vi "Weather Parse Test.vi"() -> ()   [LabVIEW 2020, in "CDM-Config.lvlib"] (continued)
eferences\": [\n                    {\n                        \"@id\": \"https://api.weather.gov/alerts/urn:oid:2.49.0.1.840.0.e016f252f56054b547b3ac73b3419f6e51da412e.001.4\",\n                        \"identifier\": \"urn:oid:2.49.0.1.840.0.e016f252f56054b547b3ac73b3419f6e51da412e.001.4\",\n                        \"sender\": \"w-nws.webmaster@noaa.gov\",\n                        \"sent\": \"2025-12-03T03:23:00-05:00\"\n                    },\n                    {\n                        \"@id\": \"https://api.weather.gov/alerts/urn:oid:2.49.0.1.840.0.e016f252f56054b547b3ac73b3419f6e51da412e.003.3\",\n                        \"identifier\": \"urn:oid:2.49.0.1.840.0.e016f252f56054b547b3ac73b3419f6e51da412e.003.3\",\n                        \"sender\": \"w-nws.webmaster@noaa.gov\",\n                        \"sent\": \"2025-12-03T03:23:00-05:00\"\n                    }\n                ],\n                \"sent\": \"2025-12-03T10:58:00-05:00\",\n                \"effective\": \"2025-12-03T10:58:00-05:00\",\n                \"onset\": \"2025-12-03T19:00:00-05:00\",\n                \"expires\": \"2025-12-03T23:00:00-05:00\",\n                \"ends\": \"2025-12-04T07:00:00-05:00\",\n                \"status\": \"Actual\",\n                \"messageType\": \"Update\",\n                \"category\": \"Met\",\n                \"severity\": \"Severe\",\n                \"certainty\": \"Likely\",\n                \"urgency\": \"Expected\",\n                \"event\": \"Heavy Freezing Spray Warning\",\n                \"sender\": \"w-nws.webmaster@noaa.gov\",\n                \"senderName\": \"NWS Marquette MI\",\n                \"headline\": \"Heavy Freezing Spray Warning issued December 3 at 10:58AM EST until December 4 at 7:00AM EST by NWS Marquette MI\",\n                \"description\": \"* WHAT...For the Gale Warning, northwest winds 25 to 30 kt with\\ngusts up to 40 kt and waves 8 to 13 ft occurring. For the\\nHeavy Freezing Spray Warning, heavy freezing spray at a rate\\nof 2 cm per hour or greater expected, and may rapidly\\naccumulate on vessels.\\n\\n* WHERE...Eagle River to Manitou Island MI, Lake Superior from\\nUpper Entrance to Portage Canal to Manitou Island MI 5NM off\\nshore to the US/Canadian Border and Lake Superior East of a\\nline from Manitou Island to Marquette MI and West of a line\\nfrom Grand Marais MI to the US/Canadian Border Beyond 5NM from\\nshore.\\n\\n* WHEN...For the Gale Warning, until 7 AM EST Thursday. For the\\nHeavy Freezing Spray Warning, from 7 PM this evening to 7 AM\\nEST Thursday.\\n\\n* IMPACTS...Operating a vessel in heavy freezing spray is\\nhazardous. Freezing spray may render mechanical and electronic\\ncomponents inoperative. Rapid ice accretion on decks and\\nsuperstructures may result in a catastrophic loss of\\nstability. Strong winds will cause hazardous waves which could\\ncapsize or damage vessels and reduce visibility.\",\n                \"instruction\": \"Mariners should prepare for dangerous accumulation of ice on\\ntheir vessel. If possible, remain in port, avoid the warning area\\nor conduct mitigation.\\n\\nMariners should alter plans to avoid these hazardous conditions.\\nRemain in port, seek safe harbor, alter course, and/or secure the\\nvessel for hazardous conditions.\",\n                \"response\": \"Avoid\",\n                \"parameters\": {\n                    \"AWIPSidentifier\": [\n                        \"MWWMQT\"\n                    ],\n                    \"WMOidentifier\": [\n                        \"WHUS73 KMQT 031558\"\n                    ],\n                    \"NWSheadline\": [\n                        \"GALE WARNING REMAINS IN EFFECT UNTIL 7 AM EST THURSDAY... ...HEAVY FREEZING SPRAY WARNING REMAINS IN EFFECT FROM 7 PM THIS EVENING TO 7 AM EST THURSDAY\"\n                    ],\n                    \"BLOCKCHANNEL\": [\n                        \"EAS\",\n                        \"NWEM\",\n                        \"CMAS\"\n                    ],\n                    \"VTEC\": [\n                        \"/O.CON.KMQT.UP.W.0017.251204T0000Z-251204T1200Z/\"\n                    ],\n                    \"eventEndingTime\": [\n                        \"2025-12-04T07:00:00-05:00\"\n                    ]\n                },\n                \"scope\": \"Public\",\n                \"code\": \"IPAWSv1.0\",\n                \"language\": \"en-US\",\n                \"web\": \"http://www.weather.gov\",\n                \"eventCode\": {\n                    \"SAME\": [\n                        \"NWS\"\n                    ],\n                    \"NationalWeatherService\": [\n                        \"UPW\"\n                    ]\n                }\n            }\n        },\n        {\n            \"id\": \"https://api.weather.gov/alerts/urn:oid:2.49.0.1.840.0.cfec64fd36b2ac790d0ebe73b8c20f8dfc3ec5cb.003.1\",\n            \"type\": \"Feature\",\n            \"geometry\": null,\n            \"properties\": {\n                \"@id\": \"https://api.weather.gov/alerts/urn:oid:2.49.0.1.840.0.cfec64fd36b2ac790d0ebe73b8c20f8dfc3ec5cb.003.1\",\n                \"@type\": \"wx:Alert\",\n                \"id\": \"urn:oid:2.49.0.1.840.0.cfec64fd36b2ac790d0ebe73b8c20f8dfc3ec5cb.003.1\",\n                \"areaDesc\": \"Black River To Ontonagon MI\",\n                \"geocode\": {\n                    \"SAME\": [\n                        \"091241\"\n                    ],\n                    \"UGC\": [\n                        \"LSZ241\"\n                    ]\n                },\n                \"affectedZones\": [\n                    \"https://api.weather.gov/zones/forecast/LSZ241\"\n                ],\n                \"references\": [\n                    {\n                        \"@id\": \"https://api.weather.gov/alerts/urn:oid:2.49.0.1.840.0.e016f252f56054b547b3ac73b3419f6e51da412e.004.1\",\n                        \"identifier\": \"urn:oid:2.49.0.1.840.0.e016f252f56054b547b3ac73b3419f6e51da412e.004.1\",\n                        \"sender\": \"w-nws.webmaster@noaa.gov\",\n                        \"sent\": \"2025-12-03T03:23:00-05:00\"\n                    }\n                ],\n                \"sent\": \"2025-12-03T10:58:00-05:00\",\n                \"effective\": \"2025-12-03T10:58:00-05:00\",\n                \"onset\": \"2025-12-03T10:58:00-05:00\",\n                \"expires\": \"2025-12-03T23:00:00-05:00\",\n                \"ends\": \"2025-12-03T16:00:00-05:00\",\n                \"status\": \"Actual\",\n                \"messageType\": \"Update\",\n                \"category\": \"Met\",\n                \"severity\": \"Minor\",\n                \"certainty\": \"Likely\",\n                \"urgency\": \"Expected\",\n                \"event\": \"Small Craft Advisory\",\n                \"sender\": \"w-nws.webmaster@noaa.gov\",\n                \"senderName\": \"NWS Marquette MI\",\n                \"headline\": \"Small Craft Advisory issued December 3 at 10:58AM EST until December 3 at 4:00PM EST by NWS Marquette MI\",\n                \"description\": \"* WHAT...For the Small Craft Advisory, northwest winds 20 to 25\\nkt with gusts up to 30 kt and waves around 7 ft occurring. For\\nthe Gale Warning, northwest winds around 25 kt with gusts up\\nto 35 kt and waves 7 to 9 ft expected.\\n\\n* WHERE...Black River to Ontonagon MI.\\n\\n* WHEN...For the Small Craft Advisory, until 4 PM EST /3 PM CST/\\nthis afternoon. For the Gale Warning, from 4 PM EST /3 PM CST/\\nthis afternoon to 1 AM EST /midnight CST/ Thursday.\\n\\n* IMPACTS...Strong winds will cause hazardous waves which could\\ncapsize or damage vessels and reduce visibility.\",\n                \"instruction\": \"Mariners should alter plans to avoid these hazardous conditions.\\nRemain in port, seek safe harbor, alter course, and/or secure the\\nvessel for hazardous conditions.\",\n                \"response\": \"Avoid\",\n                \"parameters\": {\n                    \"AWIPSidentifier\": [\n                        \"MWWMQT\"\n                    ],\n                    \"WMOidentifier\": [\n                        \"WHUS73 KMQT 031558\"\n                    ],\n                    \"NWSheadline\": [\n                        \"SMALL CRAFT ADVISORY REMAINS IN EFFECT UNTIL 4 PM EST /3 PM CST/ THIS AFTERNOON... ...GALE WARNING REMAINS IN EFFECT FROM 4 PM EST /3 PM CST/ THIS AFTERNOON TO 1 AM EST /MIDNIGHT CST/ THURSDAY\"\n                    ],\n                    \"BLOCKCHANNEL\": [\n                        \"EAS\",\n                        \"NWEM\",\n                        \"CMAS\"\n                    ],\n                    \"VTEC\": [\n                        \"/O.CON.KMQT.SC.Y.0191.000000T0000Z-251203T2100Z/\"\n                    ],\n                    \"eventEndingTime\": [\n                        \"2025-12-03T16:00:00-05:00\"\n                    ],\n                    \"expiredReferences\": [\n                        \"w-nws.webmaster@noaa.gov,urn:oid:2.49.0.1.840.0.012a713e44cf33f321dde7a7dd606454111e7dbb.001.1,2025-12-02T22:29:00-05:00 w-nws.webmaster@noaa.gov,urn:oid:2.49.0.1.840.0.74d44099106d0ecd40f7d2a62c56231069593ff3.001.1,2025-12-02T14:53:00-05:00 w-nws.webmaster@noaa.gov,urn:oid:2.49.0.1.840.0.747dd730e6a8b18ac9024c3c055a74162144c3ca.001.1,2025-12-02T10:16:00-05:00 w-nws.webmaster@noaa.gov,urn:oid:2.49.0.1.840.0.9d4c1194cc60ce916e8ebdf8581f4113872ed30b.001.1,2025-12-02T03:21:00-05:00\"\n                    ]\n                },\n                \"scope\": \"Public\",\n                \"code\": \"IPAWSv1.0\",\n                \"language\": \"en-US\",\n                \"web\": \"http://www.weather.gov\",\n                \"eventCode\": {\n                    \"SAME\": [\n                        \"NWS\"\n                    ],\n                    \"NationalWeatherService\": [\n                        \"SCY\"\n                    ]\n                }\n            }\n        },\n        {\n            \"id\": \"https://api.weather.gov/alerts/urn:oid:2.49.0.1.840.0.cfec64fd36b2ac790d0ebe73b8c20f8dfc3ec5cb.003.2\",\n            \"type\": \"Feature\",\n            \"geometry\": null,\n            \"properties\": {\n                \"@id\": \"https://api.weather.gov/alerts/urn:oid:2.49.0.1.840.0.cfec64fd36b2ac790d0ebe73b8c20f8dfc3ec5cb.003.2\",\n                \"@type\": \"wx:Alert\",\n                \"id\": \"urn:oid:2.49.0.1.840.0.cfec64fd36b2ac790d0ebe73b8c20f8dfc3ec5cb.003.2\",\n                \"areaDesc\": \"Black River To Ontonagon MI\",\n                \"geocode\": {\n                    \"SAME\": [\n                        \"091241\"\n                    ],\n                    \"UGC\": [\n                        \"LSZ241\"\n                    ]\n                },\n                \"affectedZones\": [\n                    \"https://api.weather.gov/zones/forecast/LSZ241\"\n                ],\n                \"references\": [\n                    {\n                        \"@id\": \"https://api.weather.gov/alerts/urn:oid:2.49.0.1.840.0.e016f252f56054b547b3ac73b3419f6e51da412e.004.3\",\n                        \"identifier\": \"urn:oid:2.49.0.1.840.0.e016f252f56054b547b3ac73b3419f6e51da412e.004.3\",\n                        \"sender\": \"w-nws.webmaster@noaa.gov\",\n                        \"sent\": \"2025-12-03T03:23:00-05:00\"\n                    }\n                ],\n                \"sent\": \"2025-12-03T10:58:00-05:00\",\n                \"effective\": \"2025-12-03T10:58:00-05:00\",\n                \"onset\": \"2025-12-03T16:00:00-05:00\",\n                \"expires\": \"2025-12-03T23:00:00-05:00\",\n                \"ends\": \"2025-12-04T01:00:00-05:00\",\n                \"status\": \"Actual\",\n                \"messageType\": \"Update\",\n                \"category\": \"Met\",\n                \"severity\": \"Moderate\",\n                \"certainty\": \"Likely\",\n                \"urgency\": \"Expected\",\n                \"event\": \"Gale Warning\",\n                \"sender\": \"w-nws.webmaster@noaa.gov\",\n                \"senderName\": \"NWS Marquette MI\",\n                \"headline\": \"Gale Warning issued December 3 at 10:58AM EST until December 4 at 1:00AM EST by NWS Marquette MI\",\n                \"description\": \"* WHAT...For the Small Craft Advisory, northwest winds 20 to 25\\nkt with gusts up to 30 kt and waves around 7 ft occurring. For\\nthe Gale Warning, northwest winds around 25 kt with gusts up\\nto 35 kt and waves 7 to 9 ft expected.\\n\\n* WHERE...Black River to Ontonagon MI.\\n\\n* WHEN...For the Small Craft Advisory, until 4 PM EST /3 PM CST/\\nthis afternoon. For the Gale Warning, from 4 PM EST /3 PM CST/\\nthis afternoon to 1 AM EST /midnight CST/ Thursday.\\n\\n* IMPACTS...Strong winds will cause hazardous waves which could\\ncapsize or damage vessels and reduce visibility.\",\n                \"instruction\": \"Mariners should alter plans to avoid these hazardous conditions.\\nRemain in port, seek safe harbor, alter course, and/or secure the\\nvessel for hazardous conditions.\",\n                \"response\": \"Avoid\",\n                \"parameters\": {\n                    \"AWIPSidentifier\": [\n                        \"MWWMQT\"\n                    ],\n                    \"WMOidentifier\": [\n                        \"WHUS73 KMQT 031558\"\n                    ],\n                    \"NWSheadline\": [\n                        \"SMALL CRAFT ADVISORY REMAINS IN EFFECT UNTIL 4 PM EST /3 PM CST/ THIS AFTERNOON... ...GALE WARNING REMAINS IN EFFECT FROM 4 PM EST /3 PM CST/ THIS AFTERNOON TO 1 AM EST /MIDNIGHT CST/ THURSDAY\"\n                    ],\n                    \"BLOCKCHANNEL\": [\n                        \"EAS\",\n                        \"NWEM\",\n                        \"CMAS\"\n                    ],\n                    \"VTEC\": [\n                        \"/O.CON.KMQT.GL.W.0057.251203T2100Z-251204T0600Z/\"\n                    ],\n                    \"eventEndingTime\": [\n                        \"2025-12-04T01:00:00-05:00\"\n                    ]\n                },\n                \"scope\": \"Public\",\n                \"code\": \"IPAWSv1.0\",\n                \"language\": \"en-US\",\n                \"web\": \"http://www.weather.gov\",\n                \"eventCode\": {\n                    \"SAME\": [\n                        \"NWS\"\n                    ],\n                    \"NationalWeatherService\": [\n                        \"GLW\"\n                    ]\n                }\n            }\n        },\n        {\n            \"id\": \"https://api.weather.gov/alerts/urn:oid:2.49.0.1.840.0.cfec64fd36b2ac790d0ebe73b8c20f8dfc3ec5cb.006.1\",\n            \"type\": \"Feature\",\n            \"geometry\": null,\n            \"properties\": {\n                \"@id\": \"https://api.weather.gov/alerts/urn:oid:2.49.0.1.840.0.cfec64fd36b2ac790d0ebe73b8c20f8dfc3ec5cb.006.1\",\n                \"@type\": \"wx:Alert\",\n                \"id\": \"urn:oid:2.49.0.1.840.0.cfec64fd36b2ac790d0ebe73b8c20f8dfc3ec5cb.006.1\",\n                \"areaDesc\": \"Green Bay North of line from Cedar River MI to Rock Island Passage; Seul Choix Point to Point Detour MI; 5NM East of a line from Fairport MI to Rock Island Passage\",\n                \"geocode\": {\n                    \"SAME\": [\n                        \"092221\",\n                        \"092248\",\n                        \"092250\"\n                    ],\n                    \"UGC\": [\n                        \"LMZ221\",\n                        \"LMZ248\",\n                        \"LMZ250\"\n                    ]\n                },\n                \"affectedZones\": [\n                    \"https://api.weather.gov/zones/forecast/LMZ221\",\n                    \"https://api.weather.gov/zones/forecast/LMZ248\",\n                    \"https://api.weather.gov/zones/forecast/LMZ250\"\n                ],\n                \"references\": [\n                    {\n                        \"@id\": \"https://api.weather.gov/alerts/urn:oid:2.49.0.1.840.0.e016f252f56054b547b3ac73b3419f6e51da412e.010.1\",\n                        \"identifier\": \"urn:oid:2.49.0.1.840.0.e016f252f56054b547b3ac73b3419f6e51da412e.010.1\",\n                        \"sender\": \"w-nws.webmaster@noaa.gov\",\n                        \"sent\": \"2025-12-03T03:23:00-05:00\"\n                    }\n                ],\n                \"sent\": \"2025-12-03T10:58:00-05:00\",\n                \"effective\": \"2025-12-03T10:58:00-05:00\",\n                \"onset\": \"2025-12-03T10:58:00-05:00\",\n                \"expires\": \"2025-12-03T23:00:00-05:00\",\n                \"ends\": \"2025-12-04T07:00:00-05:00\",\n                \"status\": \"Actual\",\n                \"messageType\": \"Update\",\n                \"category\": \"Met\",\n                \"severity\": \"Minor\",\n                \"certainty\": \"Likely\",\n                \"urgency\": \"Expected\",\n                \"event\": \"Small Craft Advisory\",\n                \"sender\": \"w-nws.webmaster@noaa.gov\",\n                \"senderName\": \"NWS Marquette MI\",\n                \"headline\": \"Small Craft Advisory issued December 3 at 10:58AM EST until December 4 at 7:00AM EST by NWS Marquette MI\",\n                \"description\": \"* WHAT...For the Small Craft Advisory, northwest winds 15 to 25\\nkt with gusts up to 30 kt and waves 1 to 4 ft occurring. For\\nthe Gale Watch, southwest winds 20 to 30 kt with gusts up to\\n35 kt and waves 5 to 8 ft possible.\\n\\n* WHERE...Green Bay North of line from Cedar River MI to Rock\\nIsland Passage, Seul Choix Point to Point Detour MI and 5NM\\nEast of a line from Fairport MI to Rock Island Passage.\\n\\n* WHEN...For the Small Craft Advisory, until 7 AM EST Thursday.\\nFor the Gale Watch, from Thursday evening through Friday\\nmorning.\\n\\n* IMPACTS...Strong winds can cause hazardous waves which could\\ncapsize or damage vessels and reduce visibility.\",\n                \"instruction\": \"Mariners should consider altering plans to avoid possible\\nhazardous conditions.  Remain in port, seek safe harbor, alter\\ncourse, and/or secure the vessel for severe wind and waves.\",\n                \"response\": \"Avoid\",\n                \"parameters\": {\n                    \"AWIPSidentifier\": [\n                        \"MWWMQT\"\n                    ],\n                    \"WMOidentifier\": [\n                        \"WHUS73 KMQT 031558\"\n                    ],\n                    \"NWSheadline\": [\n                        \"SMALL CRAFT ADVISORY REMAINS IN EFFECT UNTIL 7 AM EST THURSDAY... ...GALE WATCH REMAINS IN EFFECT FROM THURSDAY EVENING THROUGH FRIDAY MORNING\"\n                    ],\n                    \"BLOCKCHANNEL\": [\n                        \"EAS\",\n                        \"NWEM\",\n                        \"CMAS\"\n                    ],\n                    \"VTEC\": [\n                        \"/O.CON.KMQT.SC.Y.0191.000000T0000Z-251204T1200Z/\"\n                    ],\n                    \"eventEndingTime\": [\n                        \"2025-12-04T07:00:00-05:00\"\n                    ],\n                    \"expiredReferences\": [\n                        \"w-nws.webmaster@noaa.gov,urn:oid:2.49.0.1.840.0.012a713e44cf33f321dde7a7dd606454111e7dbb.006.1,2025-12-02T22:29:00-05:00 w-nws.webmaster@noaa.gov,urn:oid:2.49.0.1.840.0.74d44099106d0ecd40f7d2a62c56231069593ff3.006.1,2025-12-02T14:53:00-05:00 w-nws.webmaster@noaa.gov,urn:oid:2.49.0.1.840.0.747dd730e6a8b18ac9024c3c055a74162144c3ca.005.1,2025-12-02T10:16:00-05:00 w-nws.webmaster@noaa.gov,urn:oid:2.49.0.1.840.0.9d4c1194cc60ce916e8ebdf8581f4113872ed30b.003.1,2025-12-02T03:21:00-05:00\"\n                    ]\n                },\n                \"scope\": \"Public\",\n                \"code\": \"IPAWSv1.0\",\n                \"language\": \"en-US\",\n                \"web\": \"http://www.weather.gov\",\n                \"eventCode\": {\n                    \"SAME\": [\n                        \"NWS\"\n                    ],\n                    \"NationalWeatherService\": [\n                        \"SCY\"\n                    ]\n                }\n            }\n        },\n        {\n            \"id\": \"https://api.weather.gov/alerts/urn:oid:2.49.0.1.840.0.d365ea89a3273517f695e674c64a6b4737090c02.002.1\",\n            \"type\": \"Feature\",\n            \"geometry\": null,\n            \"properties\": {\n                \"@id\": \"https://api.weather.gov/alerts/urn:oid:2.49.0.1.840.0.d365ea89a3273517f695e674c64a6b4737090c02.002.1\",\n                \"@type\": \"wx:Alert\",\n                \"id\": \"urn:oid:2.49.0.1.840.0.d365ea89a3273517f695e674c64a6b4737090c02.002.1\",\n                \"areaDesc\": \"Yosemite NP outside of the valley; Upper San Joaquin River; Kaiser to Rodgers Ridge; Kings Canyon NP; Sequoia NP; South End of the Upper Sierra\",\n                \"geocode\": {\n                    \"SAME\": [\n                        \"006039\",\n                        \"006043\",\n                        \"006109\",\n                        \"006019\",\n                        \"006107\",\n                        \"006029\"\n                    ],\n                    \"UGC\": [\n                        \"CAZ323\",\n                        \"CAZ326\",\n                        \"CAZ327\",\n                        \"CAZ328\",\n                        \"CAZ330\",\n                        \"CAZ331\"\n                    ]\n                },\n                \"affectedZones\": [\n                    \"https://api.weather.gov/zones/forecast/CAZ323\",\n                    \"https://api.weather.gov/zones/forecast/CAZ326\",\n                    \"https://api.weather.gov/zones/forecast/CAZ327\",\n                    \"https://api.weather.gov/zones/forecast/CAZ328\",\n                    \"https://api.weather.gov/zones/forecast/CAZ330\",\n                    \"https://api.weather.gov/zones/forecast/CAZ331\"\n                ],\n                \"references\": [\n                    {\n                        \"@id\": \"https://api.weather.gov/alerts/urn:oid:2.49.0.1.840.0.cb9af2414be7bbb08a0146dba1918025ec85ffcc.001.1\",\n                        \"identifier\": \"urn:oid:2.49.0.1.840.0.cb9af2414be7bbb08a0146dba1918025ec85ffcc.001.1\",\n                        \"sender\": \"w-nws.webmaster@noaa.gov\",\n                        \"sent\": \"2025-12-03T05:33:00-08:00\"\n                    }\n                ],\n                \"sent\": \"2025-12-03T07:57:00-08:00\",\n                \"effective\": \"2025-12-03T07:57:00-08:00\",\n                \"onset\": \"2025-12-03T07:57:00-08:00\",\n                \"expires\": \"2025-12-03T15:00:00-08:00\",\n                \"ends\": \"2025-12-04T09:00:00-08:00\",\n                \"status\": \"Actual\",\n                \"messageType\": \"Update\",\n                \"category\": \"Met\",\n                \"severity\": \"Moderate\",\n                \"certainty\": \"Likely\",\n                \"urgency\": \"Expected\",\n                \"event\": \"Cold Weather Advisory\",\n                \"sender\": \"w-nws.webmaster@noaa.gov\",\n                \"senderName\": \"NWS Hanford CA\",\n                \"headline\": \"Cold Weather Advisory issued December 3 at 7:57AM PST until December 4 at 9:00AM PST by NWS Hanford CA\",\n                \"description\": \"* WHAT...Very cold wind chills as low as 11 below for elevations\\nabove 9000 feet.\\n\\n* WHERE...Kaiser to Rodgers Ridge, Kings Canyon NP, Sequoia NP,\\nSouth End of the Upper Sierra, Upper San Joaquin River, and\\nYosemite NP outside of the valley.\\n\\n* WHEN...Until 9 AM PST Thursday.\\n\\n* IMPACTS...The cold wind chills as low as 10 below zero could\\nresult in hypothermia if precautions are not taken. Very cold\\ntemperatures can lead to hypothermia with prolonged exposure.\",\n                \"instruction\": \"Use caution while traveling outside. Wear appropriate clothing, a\\nhat, and gloves.\",\n                \"response\": \"Prepare\",\n                \"parameters\": {\n                    \"AWIPSidentifier\": [\n                        \"NPWHNX\"\n                    ],\n                    \"WMOidentifier\": [\n                        \"WWUS76 KHNX 031557\"\n                    ],\n                    \"NWSheadline\": [\n                        \"COLD WEATHER ADVISORY REMAINS IN EFFECT UNTIL 9 AM PST THURSDAY FOR ELEVATIONS ABOVE 9000 FEET\"\n                    ],\n                    \"BLOCKCHANNEL\": [\n                        \"EAS\",\n                        \"NWEM\",\n                        \"CMAS\"\n                    ],\n                    \"VTEC\": [\n                        \"/O.CON.KHNX.CW.Y.0001.000000T0000Z-251204T1700Z/\"\n                    ],\n                    \"eventEndingTime\": [\n                        \"2025-12-04T09:00:00-08:00\"\n                    ],\n                    \"expiredReferences\": [\n                        \"w-nws.webmaster@noaa.gov,urn:oid:2.49.0.1.840.0.ef8d1d27a083b4bc8c7f3e7b074ca8ce7b49da85.002.1,2025-12-02T21:12:00-08:00 w-nws.webmaster@noaa.gov,urn:oid:2.49.0.1.840.0.22dab73e595205c33a739ef5f649c667e8025af6.002.1,2025-12-02T20:30:00-08:00 w-nws.webmaster@noaa.gov,urn:oid:2.49.0.1.840.0.404c6943eda631ddbb5686b75f29ff1b73f93377.002.1,2025-12-02T20:30:00-08:00 w-nws.webmaster@noaa.gov,urn:oid:2.49.0.1.840.0.626e22c3de1917e43dd261d699804733e982932f.001.1,2025-12-02T15:05:00-08:00 w-nws.webmaster@noaa.gov,urn:oid:2.49.0.1.840.0.7fcecc394671e4fed5feb9206c182f3bc218cad2.002.1,2025-12-02T11:48:00-08:00 w-nws.webmaster@noaa.gov,urn:oid:2.49.0.1.840.0.c2f2092361574135c2f401ab1221fc3ef8e936b9.002.1,2025-12-02T10:40:00-08:00\"\n                    ]\n                },\n                \"scope\": \"Public\",\n                \"code\": \"IPAWSv1.0\",\n                \"language\": \"en-US\",\n                \"web\": \"http://www.weather.gov\",\n                \"eventCode\": {\n                    \"SAME\": [\n                        \"NWS\"\n                    ],\n                    \"NationalWeatherService\": [\n                        \"CWY\"\n                    ]\n                }\n            }\n        },\n        {\n            \"id\": \"https://api.weather.gov/alerts/urn:oid:2.49.0.1.840.0.d365ea89a3273517f695e674c64a6b4737090c02.001.1\",\n            \"type\": \"Feature\",\n            \"geometry\": null,\n            \"properties\": {\n                \"@id\": \"https://api.weather.gov/alerts/urn:oid:2.49.0.1.840.0.d365ea89a3273517f695e674c64a6b4737090c02.001.1\",\n                \"@type\": \"wx:Alert\",\n                \"id\": \"urn:oid:2.49.0.1.840.0.d365ea89a3273517f695e674c64a6b4737090c02.001.1\",\n                \"areaDesc\": \"Grapevine\",\n                \"geocode\": {\n                    \"SAME\": [\n                        \"006029\"\n                    ],\n                    \"UGC\": [\n                        \"CAZ335\"\n                    ]\n                },\n                \"affectedZones\": [\n                    \"https://api.weather.gov/zones/forecast/CAZ335\"\n                ],\n                \"references\": [],\n                \"sent\": \"2025-12-03T07:57:00-08:00\",\n                \"effective\": \"2025-12-03T07:57:00-08:00\",\n                \"onset\": \"2025-12-03T07:57:00-08:00\",\n                \"expires\": \"2025-12-03T15:00:00-08:00\",\n                \"ends\": \"2025-12-03T15:00:00-08:00\",\n                \"status\": \"Actual\",\n                \"messageType\": \"Alert\",\n                \"category\": \"Met\",\n                \"severity\": \"Moderate\",\n                \"certainty\": \"Likely\",\n                \"urgency\": \"Expected\",\n                \"event\": \"Dense Fog Advisory\",\n                \"sender\": \"w-nws.webmaster@noaa.gov\",\n                \"senderName\": \"NWS Hanford CA\",\n                \"headline\": \"Dense Fog Advisory issued December 3 at 7:57AM PST until December 3 at 3:00PM PST by NWS Hanford CA\",\n                \"description\": \"* WHAT...Visibility one quarter mile or less in dense fog.\\n\\n* WHERE...Grapevine. This also includes Interstate 5 from Grapevine\\nup to around Ft. Tejon.\\n\\n* WHEN...Until 3 PM PST this afternoon.\\n\\n* IMPACTS...Low visibility could make driving conditions hazardous.\",\n                \"instruction\": \"If driving, slow down, use your headlights, and leave plenty of\\ndistance ahead of you.\",\n                \"response\": \"Execute\",\n                \"parameters\": {\n                    \"AWIPSidentifier\": [\n                        \"NPWHNX\"\n                    ],\n                    \"WMOidentifier\": [\n                        \"WWUS76 KHNX 031557\"\n                    ],\n                    \"NWSheadline\": [\n                        \"DENSE FOG ADVISORY IN EFFECT UNTIL 3 PM PST THIS AFTERNOON\"\n                    ],\n                    \"BLOCKCHANNEL\": [\n                        \"EAS\",\n                        \"NWEM\",\n                        \"CMAS\"\n                    ],\n                    \"VTEC\": [\n                        \"/O.EXB.KHNX.FG.Y.0035.000000T0000Z-251203T2300Z/\"\n                    ],\n                    \"eventEndingTime\": [\n                        \"2025-12-03T15:00:00-08:00\"\n                    ]\n                },\n                \"scope\": \"Public\",\n                \"code\": \"IPAWSv1.0\",\n                \"language\": \"en-US\",\n                \"web\": \"http://www.weather.gov\",\n                \"eventCode\": {\n                    \"SAME\": [\n                        \"NWS\"\n                    ],\n                    \"NationalWeatherService\": [\n                        \"FGY\"\n                    ]\n                }\n            }\n        },\n        {\n            \"id\": \"https://api.weather.gov/alerts/urn:oid:2.49.0.1.840.0.d365ea89a3273517f695e674c64a6b4737090c02.003.1\",\n            \"type\": \"Feature\",\n            \"geometry\": null,\n            \"properties\": {\n                \"@id\": \"https://api.weather.gov/alerts/urn:oid:2.49.0.1.840.0.d365ea89a3273517f695e674c64a6b4737090c02.003.1\",\n                \"@type\": \"wx:Alert\",\n                \"id\": \"urn:oid:2.49.0.1.840.0.d365ea89a3273517f695e674c64a6b4737090c02.003.1\",\n                \"areaDesc\": \"West Side of Fresno and Kings Counties; Caruthers - San Joaquin - Selma; Fresno-Clovis; Hanford - Corcoran - Lemoore; Visalia - Porterville - Reedley\",\n                \"geocode\": {\n                    \"SAME\": [\n                        \"006019\",\n                        \"006031\",\n                        \"006107\"\n                    ],\n                    \"UGC\": [\n                        \"CAZ305\",\n                        \"CAZ306\",\n                        \"CAZ307\",\n                        \"CAZ311\",\n                        \"CAZ312\"\n                    ]\n                },\n                \"affectedZones\": [\n                    \"https://api.weather.gov/zones/forecast/CAZ305\",\n                    \"https://api.weather.gov/zones/forecast/CAZ306\",\n                    \"https://api.weather.gov/zones/forecast/CAZ307\",\n                    \"https://api.weather.gov/zones/forecast/CAZ311\",\n                    \"https://api.weather.gov/zones/forecast/CAZ312\"\n                ],\n                \"references\": [\n                    {\n                        \"@id\": \"https://api.weather.gov/alerts/urn:oid:2.49.0.1.840.0.cb9af2414be7bbb08a0146dba1918025ec85ffcc.002.1\",\n                        \"identifier\": \"urn:oid:2.49.0.1.840.0.cb9af2414be7bbb08a0146dba1918025ec85ffcc.002.1\",\n                        \"sender\": \"w-nws.webmaster@noaa.gov\",\n                        \"sent\": \"2025-12-03T05:33:00-08:00\"\n                    }\n                ],\n                \"sent\": \"2025-12-03T07:57:00-08:00\",\n                \"effective\": \"2025-12-03T07:57:00-08:00\",\n                \"onset\": \"2025-12-03T07:57:00-08:00\",\n                \"expires\": \"2025-12-03T11:00:00-08:00\",\n                \"ends\": \"2025-12-03T11:00:00-08:00\",\n                \"status\": \"Actual\",\n                \"messageType\": \"Update\",\n                \"category\": \"Met\",\n                \"severity\": \"Moderate\",\n                \"certainty\": \"Likely\",\n                \"urgency\": \"Expected\",\n                \"event\": \"Dense Fog Advisory\",\n                \"sender\": \"w-nws.webmaster@noaa.gov\",\n                \"senderName\": \"NWS Hanford CA\",\n                \"headline\": \"Dense Fog Advisory issued December 3 at 7:57AM PST until December 3 at 11:00AM PST by NWS Hanford CA\",\n                \"description\": \"* WHAT...Visibility one quarter mile or less in dense fog.\\n\\n* WHERE...Caruthers - San Joaquin - Selma, Fresno-Clovis, Hanford -\\nCorcoran - Lemoore, Visalia - Porterville - Reedley, and West Side\\nof Fresno and Kings Counties.\\n\\n* WHEN...Until 11 AM PST this morning.\\n\\n* IMPACTS...Low visibility could make driving conditions hazardous.\",\n                \"instruction\": \"If driving, slow down, use your headlights, and leave plenty of\\ndistance ahead of you.\",\n                \"response\": \"Execute\",\n                \"parameters\": {\n                    \"AWIPSidentifier\": [\n                        \"NPWHNX\"\n                    ],\n                    \"WMOidentifier\": [\n                        \"WWUS76 KHNX 031557\"\n                    ],\n                    \"NWSheadline\": [\n                        \"DENSE FOG ADVISORY REMAINS IN EFFECT UNTIL 11 AM PST THIS MORNING\"\n                    ],\n                    \"BLOCKCHANNEL\": [\n                        \"EAS\",\n                        \"NWEM\",\n                        \"CMAS\"\n                    ],\n                    \"VTEC\": [\n                        \"/O.CON.KHNX.FG.Y.0035.000000T0000Z-251203T1900Z/\"\n                    ],\n                    \"eventEndingTime\": [\n                        \"2025-12-03T11:00:00-08:00\"\n                    ],\n                    \"expiredReferences\": [\n                        \"w-nws.webmaster@noaa.gov,urn:oid:2.49.0.1.840.0.ef8d1d27a083b4bc8c7f3e7b074ca8ce7b49da85.001.1,2025-12-02T21:12:00-08:00\"\n                    ]\n                },\n                \"scope\": \"Public\",\n                \"code\": \"IPAWSv1.0\",\n                \"language\": \"en-US\",\n                \"web\": \"http://www.weather.gov\",\n                \"eventCode\": {\n                    \"SAME\": [\n                        \"NWS\"\n                    ],\n                    \"NationalWeatherService\": [\n                        \"FGY\"\n                    ]\n                }\n            }\n        },\n        {\n            \"id\": \"https://api.weather.gov/alerts/urn:oid:2.49.0.1.840.0.d365ea89a3273517f695e674c64a6b4737090c02.004.1\",\n            \"type\": \"Feature\",\n            \"geometry\": null,\n            \"properties\": {\n                \"@id\": \"https://api.weather.gov/alerts/urn:oid:2.49.0.1.840.0.d365ea89a3273517f695e674c64a6b4737090c02.004.1\",\n                \"@type\": \"wx:Alert\",\n                \"id\": \"urn:oid:2.49.0.1.840.0.d365ea89a3273517f695e674c64a6b4737090c02.004.1\",\n                \"areaDesc\": \"Buttonwillow - Lost Hills - I5; Delano-Wasco-Shafter; Bakersfield; Southeast San Joaquin Valley\",\n                \"geocode\": {\n                    \"SAME\": [\n                        \"006029\",\n                        \"006031\",\n                        \"006107\"\n                    ],\n                    \"UGC\": [\n                        \"CAZ309\",\n                        \"CAZ310\",\n                        \"CAZ314\",\n                        \"CAZ315\"\n                    ]\n                },\n                \"affectedZones\": [\n                    \"https://api.weather.gov/zones/forecast/CAZ309\",\n                    \"https://api.weather.gov/zones/forecast/CAZ310\",\n                    \"https://api.weather.gov/zones/forecast/CAZ314\",\n                    \"https://api.weather.gov/zones/forecast/CAZ315\"\n                ],\n                \"references\": [\n                    {\n                        \"@id\": \"https://api.weather.gov/alerts/urn:oid:2.49.0.1.840.0.cb9af2414be7bbb08a0146dba1918025ec85ffcc.003.1\",\n                        \"identifier\": \"urn:oid:2.49.0.1.840.0.cb9af2414be7bbb08a0146dba1918025ec85ffcc.003.1\",\n                        \"sender\": \"w-nws.webmaster@noaa.gov\",\n                        \"sent\": \"2025-12-03T05:33:00-08:00\"\n                    }\n                ],\n                \"sent\": \"2025-12-03T07:57:00-08:00\",\n                \"effective\": \"2025-12-03T07:57:00-08:00\",\n                \"onset\": \"2025-12-03T07:57:00-08:00\",\n                \"expires\": \"2025-12-03T11:00:00-08:00\",\n                \"ends\": \"2025-12-03T11:00:00-08:00\",\n                \"status\": \"Actual\",\n                \"messageType\": \"Update\",\n                \"category\": \"Met\",\n                \"severity\": \"Moderate\",\n                \"certainty\": \"Likely\",\n                \"urgency\": \"Expected\",\n                \"event\": \"Dense Fog Advisory\",\n                \"sender\": \"w-nws.webmaster@noaa.gov\",\n                \"senderName\": \"NWS Hanford CA\",\n                \"headline\": \"Dense Fog Advisory issued December 3 at 7:57AM PST until December 3 at 11:00AM PST by NWS Hanford CA\",\n                \"description\": \"* WHAT...Visibility one quarter mile or less in dense fog.\\n\\n* WHERE...Bakersfield, Buttonwillow - Lost Hills - I5,\\nDelano-Wasco-Shafter, and Southeast San Joaquin Valley.\\n\\n* WHEN...Until 11 AM PST this morning.\\n\\n* IMPACTS...Low visibility could make driving conditions hazardous.\",\n                \"instruction\": \"If driving, slow down, use your headlights, and leave plenty of\\ndistance ahead of you.\",\n                \"response\": \"Execute\",\n                \"parameters\": {\n                    \"AWIPSidentifier\": [\n                        \"NPWHNX\"\n                    ],\n                    \"WMOidentifier\": [\n                        \"WWUS76 KHNX 031557\"\n                    ],\n                    \"NWSheadline\": [\n                        \"DENSE FOG ADVISORY REMAINS IN EFFECT UNTIL 11 AM PST THIS MORNING\"\n                    ],\n                    \"BLOCKCHANNEL\": [\n                        \"EAS\",\n                        \"NWEM\",\n                        \"CMAS\"\n                    ],\n                    \"VTEC\": [\n                        \"/O.CON.KHNX.FG.Y.0035.000000T0000Z-251203T1900Z/\"\n                    ],\n                    \"eventEndingTime\": [\n                        \"2025-12-03T11:00:00-08:00\"\n                    ],\n                    \"expiredReferences\": [\n                        \"w-nws.webmaster@noaa.gov,urn:oid:2.49.0.1.840.0.ef8d1d27a083b4bc8c7f3e7b074ca8ce7b49da85.003.1,2025-12-02T21:12:00-08:00 w-nws.webmaster@noaa.gov,urn:oid:2.49.0.1.840.0.22dab73e595205c33a739ef5f649c667e8025af6.001.1,2025-12-02T20:30:00-08:00 w-nws.webmaster@noaa.gov,urn:oid:2.49.0.1.840.0.404c6943eda631ddbb5686b75f29ff1b73f93377.001.1,2025-12-02T20:30:00-08:00\"\n                    ]\n                },\n                \"scope\": \"Public\",\n                \"code\": \"IPAWSv1.0\",\n                \"language\": \"en-US\",\n                \"web\": \"http://www.weather.gov\",\n                \"eventCode\": {\n                    \"SAME\": [\n                        \"NWS\"\n                    ],\n                    \"NationalWeatherService\": [\n                        \"FGY\"\n                    ]\n                }\n            }\n        },\n        {\n            \"id\": \"https://api.weather.gov/alerts/urn:oid:2.49.0.1.840.0.4a9c30a731508078f0f7520ff08e9f1f7a671578.002.1\",\n            \"type\": \"Feature\",\n            \"geometry\": null,\n            \"properties\": {\n                \"@id\": \"https://api.weather.gov/alerts/urn:oid:2.49.0.1.840.0.4a9c30a731508078f0f7520ff08e9f1f7a671578.002.1\",\n                \"@type\": \"wx:Alert\",\n                \"id\": \"urn:oid:2.49.0.1.840.0.4a9c30a731508078f0f7520ff08e9f1f7a671578.002.1\",\n                \"areaDesc\": \"Grand Portage to Grand Marais MN; Grand Marais to Taconite Harbor MN; Taconite Harbor to Silver Bay Harbor MN\",\n                \"geocode\": {\n                    \"SAME\": [\n                        \"091140\",\n                        \"091141\",\n                        \"091142\"\n                    ],\n                    \"UGC\": [\n                        \"LSZ140\",\n                        \"LSZ141\",\n                        \"LSZ142\"\n                    ]\n                },\n                \"affectedZones\": [\n                    \"https://api.weather.gov/zones/forecast/LSZ140\",\n                    \"https://api.weather.gov/zones/forecast/LSZ141\",\n                    \"https://api.weather.gov/zones/forecast/LSZ142\"\n                ],\n                \"references\": [\n                    {\n                        \"@id\": \"https://api.weather.gov/alerts/urn:oid:2.49.0.1.840.0.2b3611bf51a8d91812a27a6d34dc1646d3578776.002.1\",\n                        \"identifier\": \"urn:oid:2.49.0.1.840.0.2b3611bf51a8d91812a27a6d34dc1646d3578776.002.1\",\n                        \"sender\": \"w-nws.webmaster@noaa.gov\",\n                        \"sent\": \"2025-12-03T04:05:00-06:00\"\n                    }\n                ],\n                \"sent\": \"2025-12-03T09:55:00-06:00\",\n                \"effective\": \"2025-12-03T09:55:00-06:00\",\n                \"onset\": \"2025-12-03T09:55:00-06:00\",\n                \"expires\": \"2025-12-03T22:00:00-06:00\",\n                \"ends\": \"2025-12-04T12:00:00-06:00\",\n                \"status\": \"Actual\",\n                \"messageType\": \"Update\",\n                \"category\": \"Met\",\n                \"severity\": \"Minor\",\n                \"certainty\": \"Likely\",\n                \"urgency\": \"Expected\",\n                \"event\": \"Small Craft Advisory\",\n                \"sender\": \"w-nws.webmaster@noaa.gov\",\n                \"senderName\": \"NWS Duluth MN\",\n                \"headline\": \"Small Craft Advisory issued December 3 at 9:55AM CST until December 4 at 12:00PM CST by NWS Duluth MN\",\n                \"description\": \"* WHAT...For the Small Craft Advisory, northwest winds 10 to 20\\nkt with gusts up to 30 kt and waves 1 to 2 ft. For the Gale\\nWatch, southwest winds 15 to 25 kt with gusts up to 35 kt and\\nwaves 6 to 9 ft possible.\\n\\n* WHERE...Grand Portage to Grand Marais MN, Grand Marais to\\nTaconite Harbor MN and Taconite Harbor to Silver Bay Harbor MN.\\n\\n* WHEN...For the Small Craft Advisory, until noon CST Thursday.\\nFor the Gale Watch, from Thursday afternoon through Thursday\\nevening.\\n\\n* IMPACTS...Strong winds can cause hazardous waves which could\\ncapsize or damage vessels and reduce visibility.\\n\\n* ADDITIONAL DETAILS...Wind gusts may drop below 20 knots for a\\ntime early this morning and again Thursday morning.\",\n                \"instruction\": \"Mariners should consider altering plans to avoid possible\\nhazardous conditions.  Remain in port, seek safe harbor, alter\\ncourse, and/or secure the vessel for severe wind and waves.\",\n                \"response\": \"Avoid\",\n                \"parameters\": {\n                    \"AWIPSidentifier\": [\n                        \"MWWDLH\"\n                    ],\n                    \"WMOidentifier\": [\n                        \"WHUS73 KDLH 031555\"\n                    ],\n                    \"NWSheadline\": [\n                        \"SMALL CRAFT ADVISORY REMAINS IN EFFECT UNTIL NOON CST THURSDAY... ...GALE WATCH REMAINS IN EFFECT FROM THURSDAY AFTERNOON THROUGH THURSDAY EVENING\"\n                    ],\n                    \"BLOCKCHANNEL\": [\n                        \"EAS\",\n                        \"NWEM\",\n                        \"CMAS\"\n                    ],\n                    \"VTEC\": [\n                        \"/O.CON.KDLH.SC.Y.0132.000000T0000Z-251204T1800Z/\"\n                    ],\n                    \"eventEndingTime\": [\n                        \"2025-12-04T12:00:00-06:00\"\n                    ],\n                    \"expiredReferences\": [\n                        \"w-nws.webmaster@noaa.gov,urn:oid:2.49.0.1.840.0.04f9cf691f6928c5262dfbb988fe18619f2f30e0.002.1,2025-12-02T21:23:00-06:00 w-nws.webmaster@noaa.gov,urn:oid:2.49.0.1.840.0.d19370faedd72659268a7c7b3bafbf3617bad502.003.1,2025-12-02T15:02:00-06:00 w-nws.webmaster@noaa.gov,urn:oid:2.49.0.1.840.0.d19370faedd72659268a7c7b3bafbf3617bad502.002.1,2025-12-02T15:02:00-06:00 w-nws.webmaster@noaa.gov,urn:oid:2.49.0.1.840.0.21fbf4d0662dfb62d7facea472c0c3fe427de6a4.003.1,2025-12-02T09:49:00-06:00 w-nws.webmaster@noaa.gov,urn:oid:2.49.0.1.840.0.21fbf4d0662dfb62d7facea472c0c3fe427de6a4.001.1,2025-12-02T09:49:00-06:00 w-nws.webmaster@noaa.gov,urn:oid:2.49.0.1.840.0.a23beaf4ead8be643075481c4846f0102db9ed03.002.1,2025-12-02T02:43:00-06:00\"\n                    ]\n                },\n                \"scope\": \"Public\",\n                \"code\": \"IPAWSv1.0\",\n                \"language\": \"en-US\",\n                \"web\": \"http://www.weather.gov\",\n                \"eventCode\": {\n                    \"SAME\": [\n                        \"NWS\"\n                    ],\n                    \"NationalWeatherService\": [\n                        \"SCY\"\n                    ]\n                }\n            }\n        },\n        {\n            \"id\": \"https://api.weather.gov/alerts/urn:oid:2.49.0.1.840.0.4a9c30a731508078f0f7520ff08e9f1f7a671578.001.1\",\n            \"type\": \"Feature\",\n            \"geometry\": null,\n            \"properties\": {\n                \"@id\": \"https://api.weather.gov/alerts/urn:oid:2.49.0.1.840.0.4a9c30a731508078f0f7520ff08e9f1f7a671578.001.1\",\n                \"@type\": \"wx:Alert\",\n                \"id\": \"urn:oid:2.49.0.1.840.0.4a9c30a731508078f0f7520ff08e9f1f7a671578.001.1\",\n                \"areaDesc\": \"Outer Apostle Islands Beyond 5 NM from Mainland\",\n                \"geocode\": {\n                    \"SAME\": [\n                        \"091150\"\n                    ],\n                    \"UGC\": [\n                        \"LSZ150\"\n                    ]\n                },\n                \"affectedZones\": [\n                    \"https://api.weather.gov/zones/forecast/LSZ150\"\n                ],\n                \"references\": [\n                    {\n                        \"@id\": \"https://api.weather.gov/alerts/urn:oid:2.49.0.1.840.0.2b3611bf51a8d91812a27a6d34dc1646d3578776.001.1\",\n                        \"identifier\": \"urn:oid:2.49.0.1.840.0.2b3611bf51a8d91812a27a6d34dc1646d3578776.001.1\",\n                        \"sender\": \"w-nws.webmaster@noaa.gov\",\n                        \"sent\": \"2025-12-03T04:05:00-06:00\"\n                    }\n                ],\n                \"sent\": \"2025-12-03T09:55:00-06:00\",\n                \"effective\": \"2025-12-03T09:55:00-06:00\",\n                \"onset\": \"2025-12-03T09:55:00-06:00\",\n                \"expires\": \"2025-12-03T22:00:00-06:00\",\n                \"ends\": \"2025-12-04T12:00:00-06:00\",\n                \"status\": \"Actual\",\n                \"messageType\": \"Update\",\n                \"category\": \"Met\",\n                \"severity\": \"Minor\",\n                \"certainty\": \"Likely\",\n                \"urgency\": \"Expected\",\n                \"event\": \"Small Craft Advisory\",\n                \"sender\": \"w-nws.webmaster@noaa.gov\",\n                \"senderName\": \"NWS Duluth MN\",\n                \"headline\": \"Small Craft Advisory issued December 3 at 9:55AM CST until December 4 at 12:00PM CST by NWS Duluth MN\",\n                \"description\": \"* WHAT...For the Small Craft Advisory, northwest winds 15 to 25\\nkt with gusts up to 30 kt and waves 3 to 6 ft. For the Gale\\nWatch, southwest winds 15 to 25 kt with gusts up to 35 kt and\\nwaves 3 to 6 ft possible.\\n\\n* WHERE...Outer Apostle Islands Beyond 5 NM from Mainland.\\n\\n* WHEN...For the Small Craft Advisory, until noon CST Thursday.\\nFor the Gale Watch, from Thursday afternoon through Thursday\\nevening.\\n\\n* IMPACTS...Strong winds can cause hazardous waves which could\\ncapsize or damage vessels and reduce visibility.\\n\\n* ADDITIONAL DETAILS...Wind gusts may diminish below 20 knots\\nfor several hours early this morning and again Thursday\\nmorning.\",\n                \"instruction\": \"Mariners should consider altering plans to avoid possible\\nhazardous conditions.  Remain in port, seek safe harbor, alter\\ncourse, and/or secure the vessel for severe wind and waves.\",\n                \"response\": \"Avoid\",\n                \"parameters\": {\n                    \"AWIPSidentifier\": [\n                        \"MWWDLH\"\n                    ],\n                    \"WMOidentifier\": [\n                        \"WHUS73 KDLH 031555\"\n                    ],\n                    \"NWSheadline\": [\n                        \"SMALL CRAFT ADVISORY REMAINS IN EFFECT UNTIL NOON CST THURSDAY... ...GALE WATCH REMAINS IN EFFECT FROM THURSDAY AFTERNOON THROUGH THURSDAY EVENING\"\n                    ],\n                    \"BLOCKCHANNEL\": [\n                        \"EAS\",\n                        \"NWEM\",\n                        \"CMAS\"\n                    ],\n                    \"VTEC\": [\n                        \"/O.CON.KDLH.SC.Y.0132.000000T0000Z-251204T1800Z/\"\n                    ],\n                    \"eventEndingTime\": [\n                        \"2025-12-04T12:00:00-06:00\"\n                    ],\n                    \"expiredReferences\": [\n                        \"w-nws.webmaster@noaa.gov,urn:oid:2.49.0.1.840.0.04f9cf691f6928c5262dfbb988fe18619f2f30e0.001.1,2025-12-02T21:23:00-06:00 w-nws.webmaster@noaa.gov,urn:oid:2.49.0.1.840.0.d19370faedd72659268a7c7b3bafbf3617bad502.001.1,2025-12-02T15:02:00-06:00 w-nws.webmaster@noaa.gov,urn:oid:2.49.0.1.840.0.21fbf4d0662dfb62d7facea472c0c3fe427de6a4.002.1,2025-12-02T09:49:00-06:00 w-nws.webmaster@noaa.gov,urn:oid:2.49.0.1.840.0.a23beaf4ead8be643075481c4846f0102db9ed03.001.1,2025-12-02T02:43:00-06:00\"\n                    ]\n                },\n                \"scope\": \"Public\",\n                \"code\": \"IPAWSv1.0\",\n                \"language\": \"en-US\",\n                \"web\": \"http://www.weather.gov\",\n                \"eventCode\": {\n                    \"SAME\": [\n                        \"NWS\"\n                    ],\n                    \"NationalWeatherService\": [\n                        \"SCY\"\n                    ]\n                }\n            }\n        },\n        {\n            \"id\": \"https://api.weather.gov/alerts/urn:oid:2.49.0.1.840.0.4a9c30a731508078f0f7520ff08e9f1f7a671578.001.2\",\n            \"type\": \"Feature\",\n            \"geometry\": null,\n            \"properties\": {\n                \"@id\": \"https://api.weather.gov/alerts/urn:oid:2.49.0.1.840.0.4a9c30a731508078f0f7520ff08e9f1f7a671578.001.2\",\n                \"@type\": \"wx:Alert\",\n                \"id\": \"urn:oid:2.49.0.1.840.0.4a9c30a731508078f0f7520ff08e9f1f7a671578.001.2\",\n                \"areaDesc\": \"Outer Apostle Islands Beyond 5 NM from Mainland\",\n                \"geocode\": {\n                    \"SAME\": [\n                        \"091150\"\n                    ],\n                    \"UGC\": [\n                        \"LSZ150\"\n                    ]\n                },\n                \"affectedZones\": [\n                    \"https://api.weather.gov/zones/forecast/LSZ150\"\n                ],\n                \"references\": [\n                    {\n                        \"@id\": \"https://api.weather.gov/alerts/urn:oid:2.49.0.1.840.0.2b3611bf51a8d91812a27a6d34dc1646d3578776.001.2\",\n                        \"identifier\": \"urn:oid:2.49.0.1.840.0.2b3611bf51a8d91812a27a6d34dc1646d3578776.001.2\",\n                        \"sender\": \"w-nws.webmaster@noaa.gov\",\n                        \"sent\": \"2025-12-03T04:05:00-06:00\"\n                    }\n                ],\n                \"sent\": \"2025-12-03T09:55:00-06:00\",\n                \"effective\": \"2025-12-03T09:55:00-06:00\",\n                \"onset\": \"2025-12-04T12:00:00-06:00\",\n                \"expires\": \"2025-12-03T22:00:00-06:00\",\n                \"ends\": \"2025-12-05T00:00:00-06:00\",\n                \"status\": \"Actual\",\n                \"messageType\": \"Update\",\n                \"category\": \"Met\",\n                \"severity\": \"Moderate\",\n                \"certainty\": \"Possible\",\n                \"urgency\": \"Future\",\n                \"event\": \"Gale Watch\",\n                \"sender\": \"w-nws.webmaster@noaa.gov\",\n                \"senderName\": \"NWS Duluth MN\",\n                \"headline\": \"Gale Watch issued December 3 at 9:55AM CST until December 5 at 12:00AM CST by NWS Duluth MN\",\n                \"description\": \"* WHAT...For the Small Craft Advisory, northwest winds 15 to 25\\nkt with gusts up to 30 kt and waves 3 to 6 ft. For the Gale\\nWatch, southwest winds 15 to 25 kt with gusts up to 35 kt and\\nwaves 3 to 6 ft possible.\\n\\n* WHERE...Outer Apostle Islands Beyond 5 NM from Mainland.\\n\\n* WHEN...For the Small Craft Advisory, until noon CST Thursday.\\nFor the Gale Watch, from Thursday afternoon through Thursday\\nevening.\\n\\n* IMPACTS...Strong winds can cause hazardous waves which could\\ncapsize or damage vessels and reduce visibility.\\n\\n* ADDITIONAL DETAILS...Wind gusts may diminish below 20 knots\\nfor several hours early this morning and again Thursday\\nmorning.\",\n                \"instruction\": \"Mariners should consider altering plans to avoid possible\\nhazardous conditions.  Remain in port, seek safe harbor, alter\\ncourse, and/or secure the vessel for severe wind and waves.\",\n                \"response\": \"Prepare\",\n                \"parameters\": {\n                    \"AWIPSidentifier\": [\n                        \"MWWDLH\"\n                    ],\n                    \"WMOidentifier\": [\n                        \"WHUS73 KDLH 031555\"\n                    ],\n                    \"NWSheadline\": [\n                        \"SMALL CRAFT ADVISORY REMAINS IN EFFECT UNTIL NOON CST THURSDAY... ...GALE WATCH REMAINS IN EFFECT FROM THURSDAY AFTERNOON THROUGH THURSDAY EVENING\"\n                    ],\n                    \"BLOCKCHANNEL\": [\n                        \"EAS\",\n                        \"NWEM\",\n                        \"CMAS\"\n                    ],\n                    \"VTEC\": [\n                        \"/O.CON.KDLH.GL.A.0018.251204T1800Z-251205T0600Z/\"\n                    ],\n                    \"eventEndingTime\": [\n                        \"2025-12-05T00:00:00-06:00\"\n                    ],\n                    \"expiredReferences\": [\n                        \"w-nws.webmaster@noaa.gov,urn:oid:2.49.0.1.840.0.04f9cf691f6928c5262dfbb988fe18619f2f30e0.001.2,2025-12-02T21:23:00-06:00\"\n                    ]\n                },\n                \"scope\": \"Public\",\n                \"code\": \"IPAWSv1.0\",\n                \"language\": \"en-US\",\n                \"web\": \"http://www.weather.gov\",\n                \"eventCode\": {\n                    \"SAME\": [\n                        \"NWS\"\n                    ],\n                    \"NationalWeatherService\": [\n                        \"GLA\"\n                    ]\n                }\n            }\n        },\n        {\n            \"id\": \"https://api.weather.gov/alerts/urn:oid:2.49.0.1.840.0.4a9c30a731508078f0f7520ff08e9f1f7a671578.003.1\",\n            \"type\": \"Feature\",\n            \"geometry\": null,\n            \"properties\": {\n                \"@id\": \"https://api.weather.gov/alerts/urn:oid:2.49.0.1.840.0.4a9c30a731508078f0f7520ff08e9f1f7a671578.003.1\",\n                \"@type\": \"wx:Alert\",\n                \"id\": \"urn:oid:2.49.0.1.840.0.4a9c30a731508078f0f7520ff08e9f1f7a671578.003.1\",\n                \"areaDesc\": \"Silver Bay Harbor to Two Harbors MN; Two Harbors to Duluth MN\",\n                \"geocode\": {\n                    \"SAME\": [\n                        \"091143\",\n                        \"091144\"\n                    ],\n                    \"UGC\": [\n                        \"LSZ143\",\n                        \"LSZ144\"\n                    ]\n                },\n                \"affectedZones\": [\n                    \"https://api.weather.gov/zones/forecast/LSZ143\",\n                    \"https://api.weather.gov/zones/forecast/LSZ144\"\n                ],\n                \"references\": [\n                    {\n                        \"@id\": \"https://api.weather.gov/alerts/urn:oid:2.49.0.1.840.0.2b3611bf51a8d91812a27a6d34dc1646d3578776.003.1\",\n                        \"identifier\": \"urn:oid:2.49.0.1.840.0.2b3611bf51a8d91812a27a6d34dc1646d3578776.003.1\",\n                        \"sender\": \"w-nws.webmaster@noaa.gov\",\n                        \"sent\": \"2025-12-03T04:05:00-06:00\"\n                    }\n                ],\n                \"sent\": \"2025-12-03T09:55:00-06:00\",\n                \"effective\": \"2025-12-03T09:55:00-06:00\",\n                \"onset\": \"2025-12-03T09:55:00-06:00\",\n                \"expires\": \"2025-12-03T22:00:00-06:00\",\n                \"ends\": \"2025-12-04T12:00:00-06:00\",\n                \"status\": \"Actual\",\n                \"messageType\": \"Update\",\n                \"category\": \"Met\",\n                \"severity\": \"Minor\",\n                \"certainty\": \"Likely\",\n                \"urgency\": \"Expected\",\n                \"event\": \"Small Craft Advisory\",\n                \"sender\": \"w-nws.webmaster@noaa.gov\",\n                \"senderName\": \"NWS Duluth MN\",\n                \"headline\": \"Small Craft Advisory issued December 3 at 9:55AM CST until December 4 at 12:00PM CST by NWS Duluth MN\",\n                \"description\": \"* WHAT...For the Small Craft Advisory, west winds 10 to 20 kt\\nwith gusts up to 25 kt and waves 1 to 2 ft. For the Gale\\nWatch, southwest winds 15 to 25 kt with gusts up to 35 kt and\\nwaves 3 to 6 ft possible.\\n\\n* WHERE...Silver Bay Harbor to Two Harbors MN and Two Harbors to\\nDuluth MN.\\n\\n* WHEN...For the Small Craft Advisory, until noon CST Thursday.\\nFor the Gale Watch, from Thursday afternoon through Thursday\\nevening.\\n\\n* IMPACTS...Strong winds can cause hazardous waves which could\\ncapsize or damage vessels and reduce visibility.\\n\\n* ADDITIONAL DETAILS...Wind gusts may drop below 20 knots for a\\ntime early this morning and again Thursday morning.\",\n                \"instruction\": \"Mariners should consider altering plans to avoid possible\\nhazardous conditions.  Remain in port, seek safe harbor, alter\\ncourse, and/or secure the vessel for severe wind and waves.\",\n                \"response\": \"Avoid\",\n                \"parameters\": {\n                    \"AWIPSidentifier\": [\n                        \"MWWDLH\"\n                    ],\n                    \"WMOidentifier\": [\n                        \"WHUS73 KDLH 031555\"\n                    ],\n                    \"NWSheadline\": [\n                        \"SMALL CRAFT ADVISORY REMAINS IN EFFECT UNTIL NOON CST THURSDAY... ...GALE WATCH REMAINS IN EFFECT FROM THURSDAY AFTERNOON THROUGH THURSDAY EVENING\"\n                    ],\n                    \"BLOCKCHANNEL\": [\n                        \"EAS\",\n                        \"NWEM\",\n  
